vi "Write Filter.vi"(8 "error in (no error)":errorcluster, 10 "Filter":T1 {"Deny List (ID)" format="%.0x"; "Allow List (ID)" format="%.0x"}, 11 "CAN_Logic in":refnum<class "CAN_Logic.lvclass">) -> (0 "error out":errorcluster, 3 "CAN_Logic out":refnum<class "CAN_Logic.lvclass">)   [LabVIEW 2021, in "CAN_Logic.lvclass"]
uses:
  CAN_Logic.lvclass
  CAN_Logic.lvclass/CAN_Logic.ctl
  typedef/CAN Filter.ctl
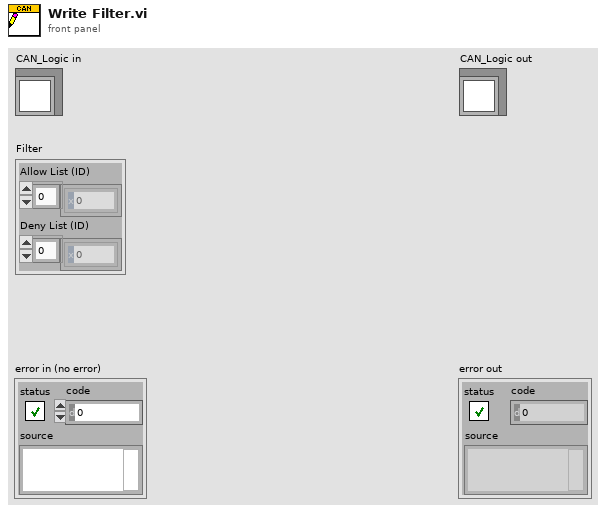
[diagram p1: front panel]
types:
  T1 = typedef "CAN_Logic.lvclass/CAN Filter.ctl" = cluster{"Allow List (ID)":u32[], "Deny List (ID)":u32[]}
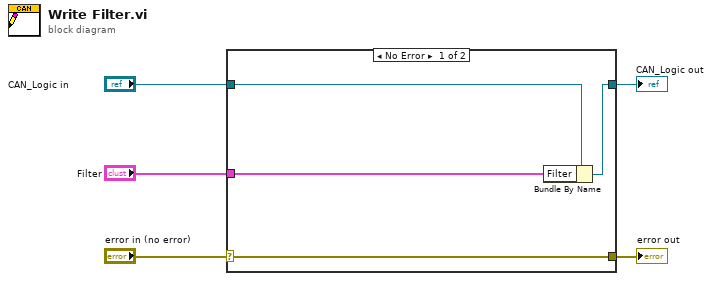
[diagram p0: block diagram]
diagram:
  n1 = case shown="No Error" "error in (no error)" {
    selector: "error in (no error)" -> [w9 w10]
    tunnel: [w9 w10] -> w4
    tunnel: [w7 w11] -> w2
    tunnel: "CAN_Logic in" -> [w8 w11]
    tunnel: "Filter" -> [w6 _]
    frame No Error {
      n2 = Bundle By Name(cluster=w8, "Filter"=w6) -> (w7:refnum<class "CAN_Logic.lvclass">)
    }
    frame Error {
    }
  }
  "error out" <- w4
  "CAN_Logic out" <- w2
